vi "Voltage and Current Ring Chooser.vi"(8 "error in (no error)":errorcluster, 11 "Tektronix PA1000 in":refnum<class "Tektronix PA1000.lvclass">) -> (0 "error out":errorcluster, 3 "Tektronix PA1000 out":refnum<class "Tektronix PA1000.lvclass">)   [LabVIEW 2014, in "Generic Power Analyzer.lvlib" / "Tektronix PA1000.lvlib" / "Tektronix PA1000.lvclass"]
uses:
  Tektronix PA1000.lvclass
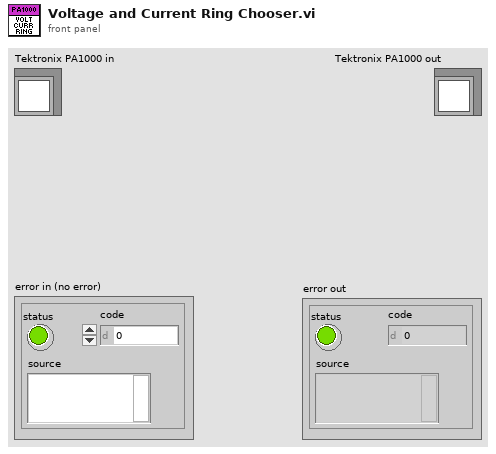
[diagram p1: front panel]
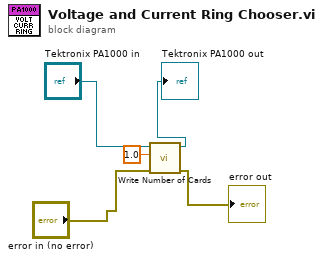
[diagram p0: block diagram]
diagram:
  n1 = call-dynamic "Write Number of Cards.vi"("error in (no error)"="error in (no error)", "Number of Cards"=1.0, "Generic Instrument in"="Tektronix PA1000 in") -> ("error out"=→"error out":errorcluster, "Generic Instrument out"=→"Tektronix PA1000 out":refnum<class "Tektronix PA1000.lvclass">)  [unwired: 7 in]
